vi "Bessel Function Yv.vi"(2 "v":dbl format="%.2f", 3 "x":dbl format="%.2f") -> (1 "Yv(x)":dbl format="%.2f")   [LabVIEW 2014, in "NI_Gmath.lvlib"]
doc: "Computes the Bessel function of the second kind, also known as the Neumann function."
uses:
  NI_Gmath.lvlib
  lvanlys.dll
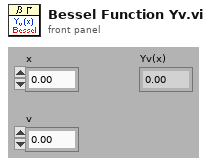
[diagram p1: front panel]
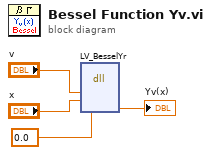
[diagram p0: block diagram]
diagram:
  n1 = dll-call lib="C:/Program Files (x86)/National Instruments/LabVIEW 2014/resource/lvanlys.*" fn="LV_BesselYr"("v"="v", "x"="x", "Yv(x)"=0.0 ("Jr")) -> ("Yv(x)"=→"Yv(x)":dbl)  [unwired: 6 in, 2 out]
